vi "LVClass_CorrectionDataManager GetActuatorInluence.vi"(0 "CorrectionDataManager in":refnum<class "CorrectionDataManager.lvclass">, 5 "N° actuator":i32, 7 "Use actuator pupil ?":bool, 9 "Influence HasoSlopes":refnum<class "HasoSlopes.lvclass">, 11 "error in (no error)":errorcluster) -> (4 "CorrectionDataManager out":refnum<class "CorrectionDataManager.lvclass">, 10 "Influence HasoSlopes (dup)":refnum<class "HasoSlopes.lvclass">, 15 "error out":errorcluster)   [LabVIEW 2020, in "CorrectionDataManager.lvclass"]
doc: "Get actuator influence as HasoSlopes.\n\n<B>corrdata_managerIn</B> : CorrDataManager object.\n<B>corrdata_managerOut</B> : CorrDataManager object.\n<B>actuator_index</B> : Actuator index.\n<B>use_actuator_pupil</B> : If true, influence pupil will be the actuator's one, else it will be the\n corrdata_manager one.\n<B>influence</B> : HasoSlopes or Phase object, representing the actuator influence.\n<B>is_phase</B> : define if influence container is a HasoSlopes or Phase."
uses:
  CorrectionDataManager.lvclass
  HasoSlopes/HasoSlopes.lvclass
  CorrectionDataManager.lvclass/CorrectionDataManager.ctl
  HasoSlopes/LVClass_HasoSlopes Read HasoSlopes _ property.vi
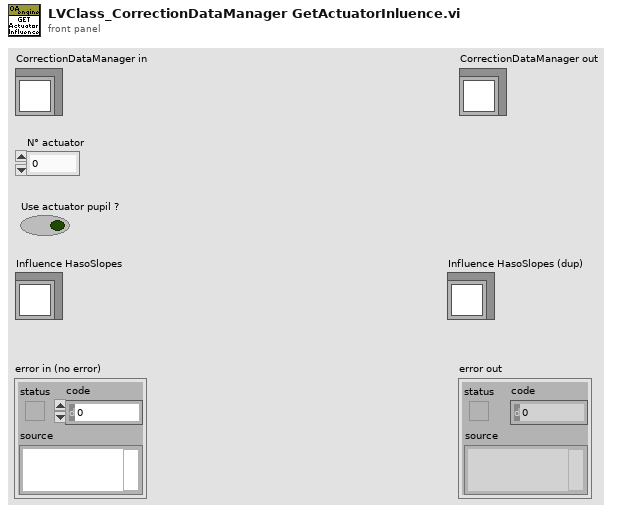
[diagram p1: front panel]
types:
  T1 = typedef "ClassID.ctl" = i64
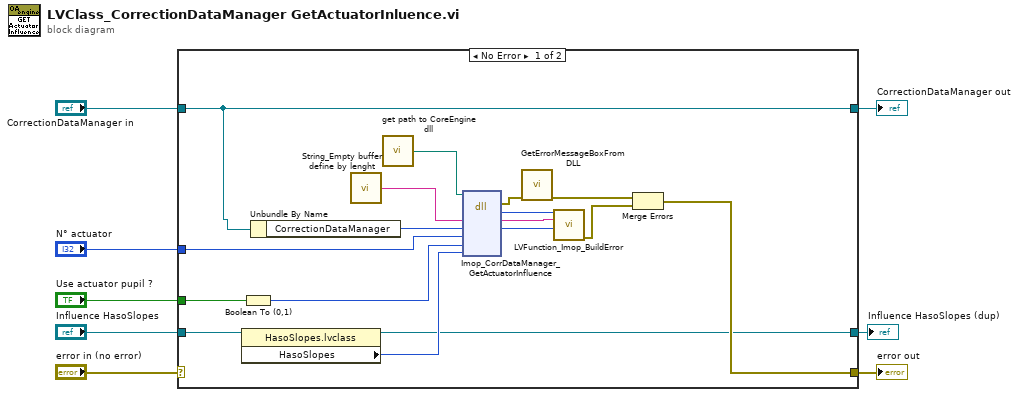
[diagram p0: block diagram]
diagram:
  n1 = case shown="No Error" "error in (no error)" {
    selector: "error in (no error)" -> [_ w28]
    tunnel: [w18 w28] -> w8
    tunnel: [w16 w27] -> w7
    tunnel: "CorrectionDataManager in" -> [w16 w27]
    tunnel: "N° actuator" -> [w15 _]
    tunnel: "Use actuator pupil ?" -> [w12 _]
    tunnel: "Influence HasoSlopes" -> [w14 w26]
    tunnel: [w10 w26] -> w1
    frame No Error {
      n2 = property class="HasoSlopes.lvclass"(reference=w14) -> (reference out=w10:refnum<class "HasoSlopes.lvclass">, "HasoSlopes"=w13:T1)  [unwired: 1 in, 1 out]
      n3 = Boolean To (0,1)(Boolean=w12) -> (0, 1=w11:i16)
      n4 = Unbundle By Name(w16) -> ("CorrectionDataManager"=w17:T1)
      n5 = call "String_Empty buffer define by lenght.vi"() -> ("Empty buffer"=w23:string)  [unwired: 1 in]
      n6 = call "get path to CoreEngine dll.vi"() -> ("path to wavekit library"=w22:path)  [unwired: 14 in, 1 out]
      n7 = dll-call lib="D:/FLE/0.Code/CoreEngine4_Suite/LV2011_interface/DLLs/c_interface_vc100.dll" fn="Imop_CorrDataManager_GetActuatorInfluence"(path in=w22, "message"=w23, "corrdata_manager"=w17, "experience_index"=w15, "Use actuator Pupil"=w11, "Influence HasoSlopes"=w13) -> (error out=w21:errorcluster, "return type"=w25:i32, "message"=w24:string, "corrdata_manager"=w9:i64)  [unwired: 5 in, 1 out]
      n8 = call "GetErrorMessageBoxFromDLL.vi"("error IN"=w21) -> ("error OUT"=w20:errorcluster)  [unwired: 10 in]
      n9 = call "LVFunction_Imop_BuildError.vi"("code"=w25, "String to Prepend to source (\"\")"=w24, "Adresse"=w9) -> ("error out"=w19:errorcluster)  [unwired: 12 in]
      n10 = Merge Errors(w20, w19) -> (w18:errorcluster)
    }
    frame Error {
    }
  }
  "error out" <- w8
  "CorrectionDataManager out" <- w7
  "Influence HasoSlopes (dup)" <- w1
